vi "Child Inheritance.vi"(8 "error in (no error)":errorcluster, 10 "Child In":refnum<class "Circular Buffer.lvclass">, 11 "Parent In":refnum<class "Circular Buffer 2D U16 DVR Queue Circular Buffer.lvclass">) -> (0 "error out":errorcluster, 2 "Child Out":refnum<class "Circular Buffer.lvclass">, 3 "Parent Out":refnum<class "Circular Buffer 2D U16 DVR Queue Circular Buffer.lvclass">)   [LabVIEW 2024, in "Circular Buffer 2D U16 DVR Queue Circular Buffer.lvclass"]
uses:
  Circular Buffer 2D U16 DVR Queue Circular Buffer.lvclass
  Ancestor Class/Circular Buffer/Circular Buffer.lvclass
  Circular Buffer 2D U16 DVR Queue Circular Buffer.lvclass/Circular Buffer 2D U16 DVR Queue Circular Buffer.ctl
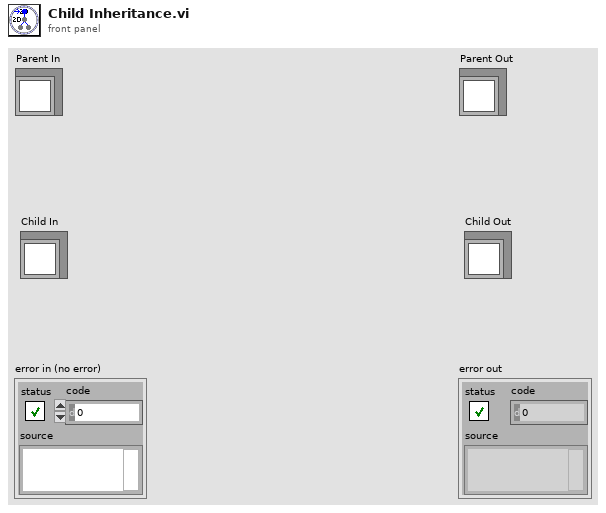
[diagram p1: front panel]
types:
  T1 = typedef "2D U16 DVR Queue.ctl" = refnum<queue>
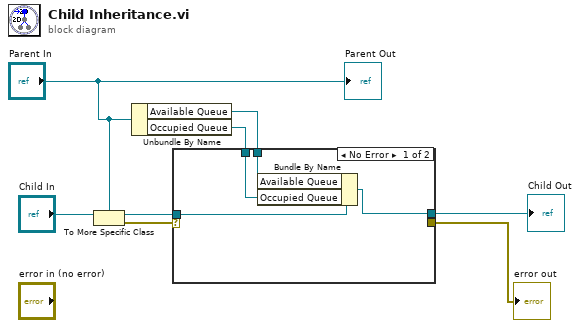
[diagram p0: block diagram]
diagram:
  n1 = To More Specific Class(target class="Parent In", reference="Child In") -> (specific class reference=w5:refnum<class "Circular Buffer 2D U16 DVR Queue Circular Buffer.lvclass">, error out=w6:errorcluster)  [unwired: 1 in]
  n2 = Unbundle By Name("Parent In") -> ("Available Queue"=w4:T1, "Occupied Queue"=w3:T1)
  n3 = case shown="No Error" w6 {
    selector: w6 -> [_ w13]
    tunnel: w5 -> [w12 w14]
    tunnel: w4 -> [w11 _]
    tunnel: w3 -> [w10 _]
    tunnel: [w9 w14] -> w2
    tunnel: [_ w13] -> w1
    frame No Error {
      n4 = Bundle By Name(cluster=w12, "Available Queue"=w11, "Occupied Queue"=w10) -> (w9:refnum<class "Circular Buffer 2D U16 DVR Queue Circular Buffer.lvclass">)
    }
    frame Error {
    }
  }
  "error out" <- w1
  "Child Out" <- w2
  "Parent Out" <- "Parent In"
